vi "tablePopulation.vi"(6 "Table Control":string[][](table), 8 "new element/subarray":string[](array[string]), 11 "Numeric":dbl) -> (0 "dimension size":i32=2, 1 "Numeric 2":dbl, 3 "output array":string[][](array[string]))   [LabVIEW 2018]
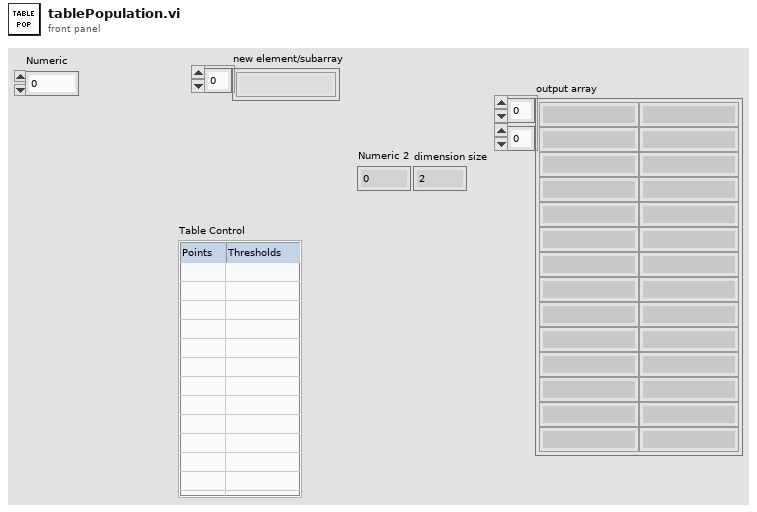
[diagram p1: front panel]
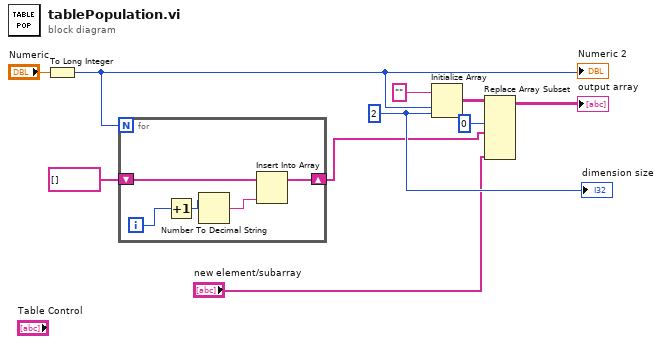
[diagram p0: block diagram]
diagram:
  w6 = 2 ("dimension size")
  n1 = To Long Integer(number="Numeric") -> (32bit integer=w1:i32)
  "Numeric 2" <- w1
  n2 = for {
    N: w1 -> [_]
    shift-right: [w11] -> w4
    shift-left: string[] [] -> [w12]
    i -> [w13]
    n3 = Increment(x=w13) -> (x+1=w14:i32)
    n4 = Number To Decimal String(number=w14) -> (decimal integer string=w15:string)  [unwired: 1 in]
    n5 = Insert Into Array(array=w12, new element=w15) -> (w11:string[])  [unwired: 1 in]
  }
  n6 = Initialize Array("", w1, w6) -> (w8:string[][])
  n7 = Replace Array Subset(array=w8, new element #1=w4, index (col) #1=0 ("disabled index (col)"), new element #2="new element/subarray") -> (→"output array":string[][])  [unwired: 3 in]
  "dimension size" <- w6
